vi "Persist New Entity.vi"(8 "error in (no error)":errorcluster, 9 "Entity":refnum<class "Entity.lvclass">, 10 "Types":refnum<class "Type.lvclass">[](array[class]), 11 "Database in":refnum<class "Dummy DB.lvclass">) -> (0 "error out":errorcluster, 2 "New ID":T1, 3 "Database out":refnum<class "Dummy DB.lvclass">)   [LabVIEW 2020, in "Scratchpad.lvlib" / "Dummy DB.lvclass"]
uses:
  Dummy DB.lvclass
  Conditum/Entity/Entity.lvclass
  Conditum/Entity ID.ctl
  Conditum/Columns/Type/Type.lvclass
  Conditum/Conditum.lvlib
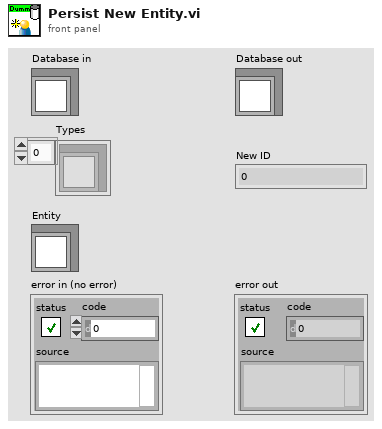
[diagram p1: front panel]
types:
  T1 = typedef "Conditum.lvlib/Entity ID.ctl" = i64
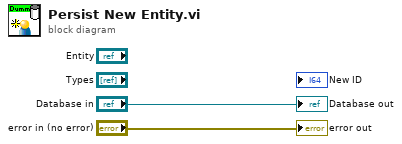
[diagram p0: block diagram]
diagram:
  "error out" <- "error in (no error)"
  "Database out" <- "Database in"
